vi "SDCP SMF Receiver and Transmitter - Read Trace File Updated.vi"() -> ()   [LabVIEW 2020]
uses:
  <vilib>/Utility/file.llb/Read Delimited Spreadsheet (string).vi
panel:
  out "error out":errorcluster
  in  "error in (no error)":errorcluster
  in  "Trace File Path":path=path "E:/Projects/System Diagnostics and Control Protocol/SDCP_LabVIEW/temp/Trace Files/21 Apr 2024 16-09.csv"
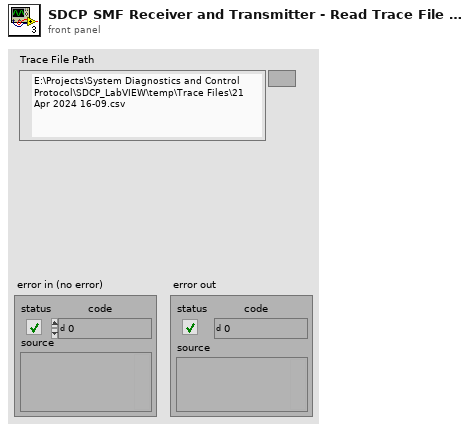
[diagram p1: front panel]
types:
  T1 = cluster{"Data bytes":u8[], "Time (ms)":dbl, "Frame ID":i32}
  T2 = cluster{"Data bytes":u8[], "Time (ms)":dbl, "Frame ID":i32}[]
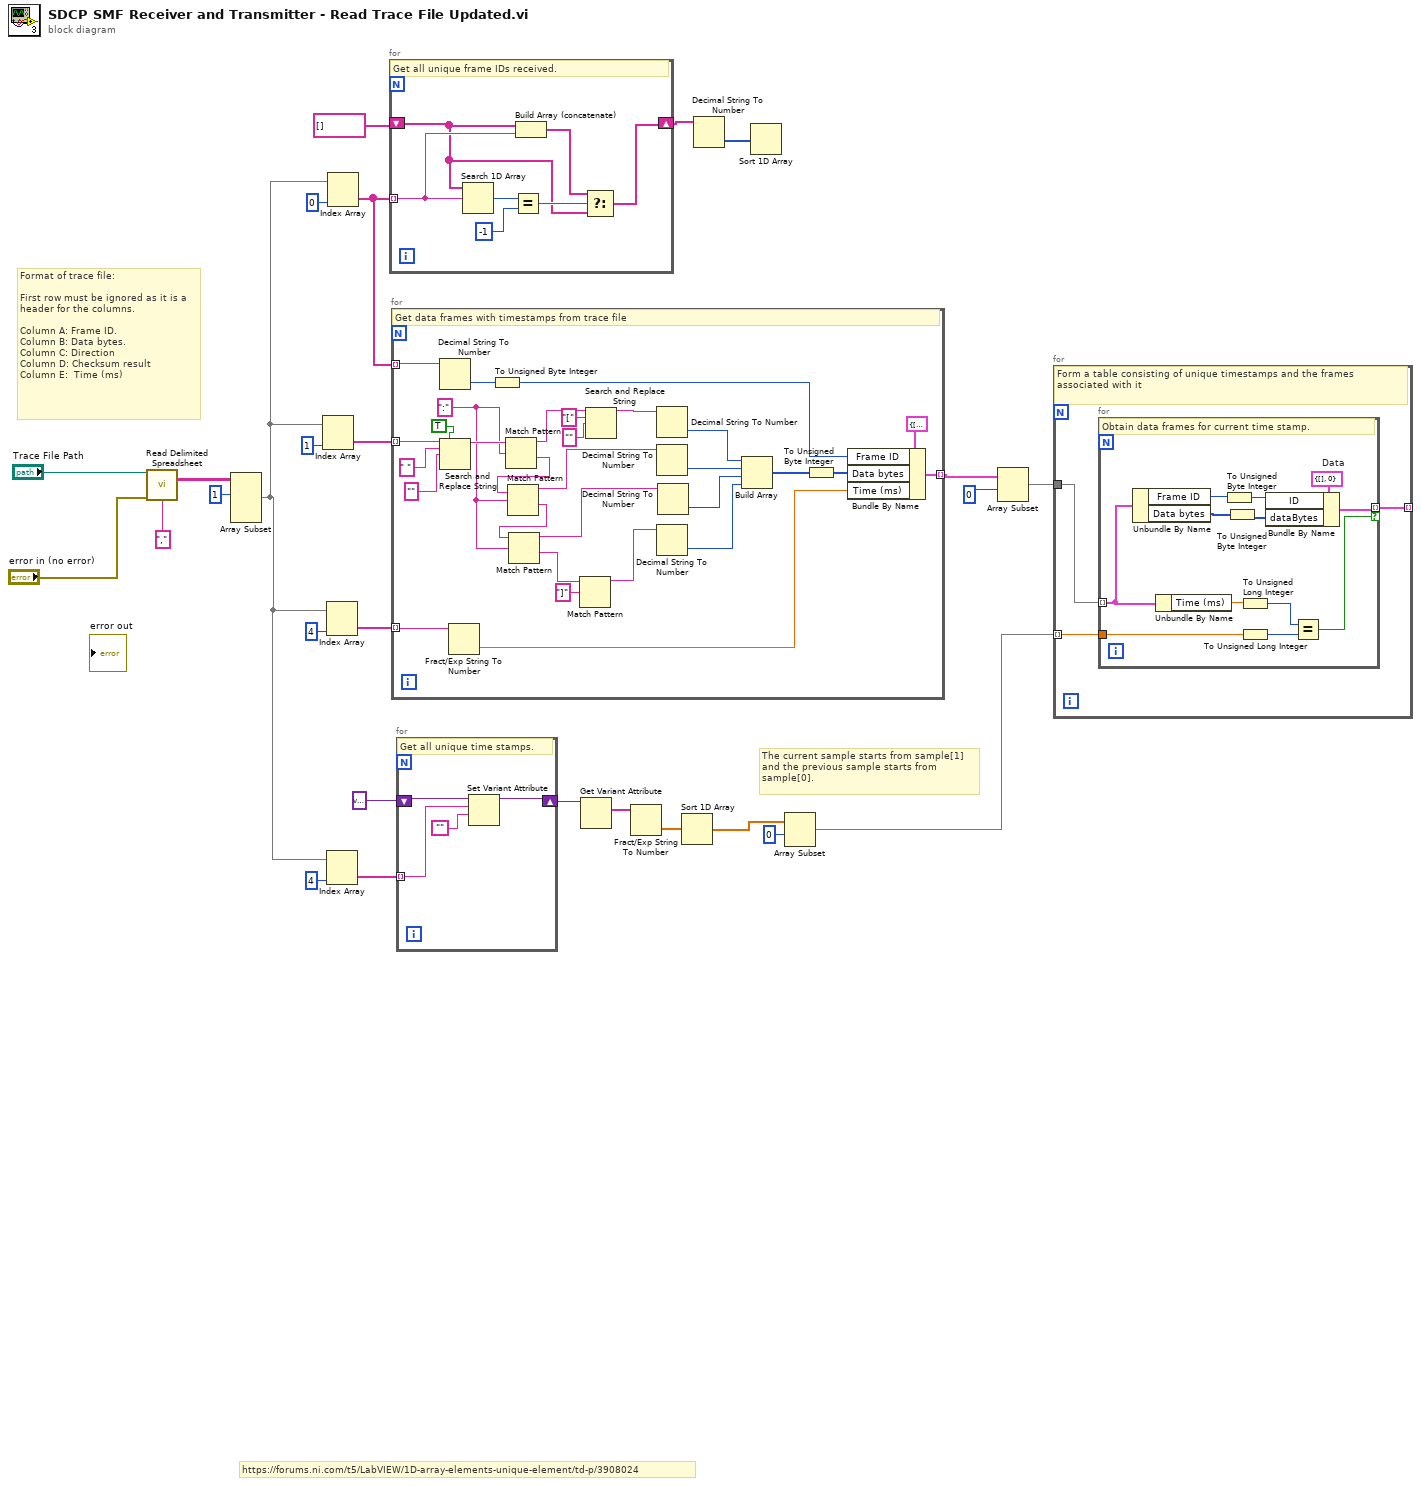
[diagram p0: block diagram]
diagram:
  # "The current sample starts from sample[1]\nand the previous sample starts from \nsample[0]."
  # "https://forums.ni.com/t5/LabVIEW/1D-array-elements-unique-element/td-p/3908024"
  # "Format of trace file:\n\nFirst row must be ignored as it is a\nheader for the columns.\n\nColumn A: Frame ID.\nColumn B: Data bytes.\nColumn C: Direction\nColumn D: Checksum result\nColumn E:  Time (ms)"
  n1 = call-poly <vilib>:"Read Delimited Spreadsheet.vi"("file path (dialog if empty)"="Trace File Path", "error in (no error)"="error in (no error)", "delimiter (\\t)"="," ("delimiter (\\t)")) -> ("all rows"=w23:string[][])  [unwired: 7 in, 5 out]
  n2 = Array Subset(array=w23, index (row)=1 ("index")) -> (w11:string[][])  [unwired: 3 in]
  n3 = Index Array(array=w11, index (col)=1 ("disabled index (col)")) -> (element=w17:string[])  [unwired: 1 in]
  n4 = Index Array(array=w11, index (col)=4 ("disabled index (col)")) -> (element=w15:string[])  [unwired: 1 in]
  n5 = Index Array(array=w11, index (col)=4 ("disabled index (col)")) -> (element=w12:string[])  [unwired: 1 in]
  n6 = Index Array(array=w11, index (col)=0 ("disabled index (col)")) -> (element=w14:string[])  [unwired: 1 in]
  n7 = for {
    tunnel: w14 -> [w31] mode=indexing
    shift-right: [w28] -> w20
    shift-left: string[] [] -> [w29]
    # "Get all unique frame IDs received."
    n8 = Search 1D Array(1D array=w29, element=w31) -> (index of element=w34:i32)  [unwired: 1 in]
    n9 = Equal?(x=w34, y=-1) -> (x = y?=w32:bool)
    n10 = Build Array (concatenate)(w29, w31) -> (w30:string[])
    n11 = Select(t=w30, s=w32, f=w29) -> (s? t:f=w28:string[])
  }
  n12 = for {
    tunnel: w17 -> [w44] mode=indexing
    tunnel: w15 -> [w40] mode=indexing
    tunnel: [w38] -> w1 mode=indexing
    tunnel: w14 -> [w37] mode=indexing
    w48 = ":" ("regular expression")
    # "Get data frames with timestamps from trace file"
    n13 = Decimal String To Number(string=w37) -> (number=w36:i32)  [unwired: 2 in, 1 out]
    n14 = Search and Replace String(replace all?=TRUE ("replace all? (F)"), input string=w44, search string=" ", replace string="" ("replace string (\"\")")) -> (result string=w52:string)  [unwired: 4 in, 3 out]
    n15 = Fract/Exp String To Number(string=w40) -> (number=w39:dbl)  [unwired: 3 in, 1 out]
    n16 = To Unsigned Byte Integer(number=w36) -> (unsigned 8bit integer=w35:u8)
    n17 = Match Pattern(string=w52, regular expression=w48) -> (before substring=w63:string, after substring=w53:string)  [unwired: 1 in, 2 out]
    n18 = Match Pattern(string=w53, regular expression=w48) -> (before substring=w56:string, after substring=w54:string)  [unwired: 1 in, 2 out]
    n19 = Match Pattern(string=w54, regular expression=w48) -> (before substring=w57:string, after substring=w55:string)  [unwired: 1 in, 2 out]
    n20 = Match Pattern(string=w55, regular expression="]") -> (before substring=w58:string)  [unwired: 1 in, 3 out]
    n21 = Search and Replace String(input string=w63, search string="[", replace string="" ("replace string (\"\")")) -> (result string=w64:string)  [unwired: 5 in, 3 out]
    n22 = Decimal String To Number(string=w64) -> (number=w59:i32)  [unwired: 2 in, 1 out]
    n23 = Decimal String To Number(string=w56) -> (number=w60:i32)  [unwired: 2 in, 1 out]
    n24 = Decimal String To Number(string=w58) -> (number=w62:i32)  [unwired: 2 in, 1 out]
    n25 = Decimal String To Number(string=w57) -> (number=w61:i32)  [unwired: 2 in, 1 out]
    n26 = Build Array(w59, w60, w61, w62) -> (w42:i32[])
    n27 = To Unsigned Byte Integer(number=w42) -> (unsigned 8bit integer=w41:u8[])
    n28 = Bundle By Name(cluster=T1 {"Data bytes"=[], "Time (ms)"=0.0, "Frame ID"=0}, "Frame ID"=w35, "Data bytes"=w41, "Time (ms)"=w39) -> (w38:T1)
  }
  n29 = for {
    tunnel: w12 -> [w66] mode=indexing
    shift-right: [w67] -> w9
    shift-left: variant -> [w68]
    # "Get all unique time stamps."
    n30 = Set Variant Attribute(Variant=w68, name=w66, value="") -> (Variant out=w67:variant)  [unwired: 1 in, 2 out]
  }
  n31 = Get Variant Attribute(Variant=w9) -> (names=w8:string[])  [unwired: 3 in, 3 out]
  n32 = Fract/Exp String To Number(string=w8) -> (number=w7:dbl[])  [unwired: 3 in, 1 out]
  n33 = Sort 1D Array(array=w7) -> (sorted array=w2:dbl[])
  n34 = Decimal String To Number(string=w20) -> (number=w19:i32[])  [unwired: 2 in, 1 out]
  n35 = Sort 1D Array(array=w19) -> ()  [unwired: 1 out]
  n36 = Array Subset(array=w2, index=0) -> (w6:dbl[])  [unwired: 1 in]
  n37 = Array Subset(array=w1, index=0) -> (w4:T2)  [unwired: 1 in]
  n38 = for {
    tunnel: w6 -> [w70] mode=indexing
    tunnel: w4 -> [w71]
    tunnel: [w69] -> _ mode=indexing
    # "Form a table consisting of unique timestamps and the frames associated with it"
    n39 = for {
      tunnel: w70 -> [w82]
      tunnel: w71 -> [w79] mode=indexing
      tunnel: [w72] -> w69 mode=indexing if=w76
      w75 = cluster{"dataBytes":u8[], "ID":i32} {"dataBytes"=[], "ID"=0}  # Data
      # "Obtain data frames for current time stamp."
      n40 = Unbundle By Name(w79) -> ("Frame ID"=w78:i32, "Data bytes"=w77:u8[])
      n41 = Unbundle By Name(w79) -> ("Time (ms)"=w83:dbl)
      n42 = To Unsigned Byte Integer(number=w78) -> (unsigned 8bit integer=w74:u8)
      n43 = To Unsigned Byte Integer(number=w77) -> (unsigned 8bit integer=w73:u8[])
      n44 = To Unsigned Long Integer(number=w83) -> (unsigned 32bit integer=w81:u32)
      n45 = To Unsigned Long Integer(number=w82) -> (unsigned 32bit integer=w80:u32)
      n46 = Bundle By Name(cluster=w75, "ID"=w74, "dataBytes"=w73) -> (w72:cluster{"dataBytes":u8[], "ID":i32})
      n47 = Equal?(x=w81, y=w80) -> (x = y?=w76:bool)
    }
  }
